vi "dfd_Cast Vector Size.vi"(1 "expected size":i32, 2 "vector in":dbl[](array[numeric]) format="%.2f") -> (0 "vector out":dbl[](array[numeric]) format="%.2f")   [LabVIEW 2017, in "NI_DigFilterLicensed.lvlib"]
uses:
  <vilib>/addons/Digital Filter Design/NI_DigFilterLicensed.lvlib
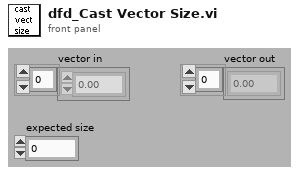
[diagram p1: front panel]
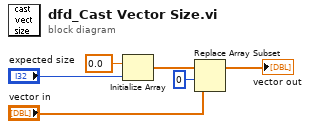
[diagram p0: block diagram]
diagram:
  n1 = Initialize Array(0.0 ("element"), "expected size") -> (w4:dbl[])
  n2 = Replace Array Subset(array=w4, new element="vector in", index=0) -> (→"vector out":dbl[])
